vi "WIMDA data insert.vi"(8 "error in (no error)":errorcluster, 11 "WIMDA-data":T1) -> (0 "error out":errorcluster)   [LabVIEW 2016, in "AIRMAR WeatherCaster.lvlib"]
uses:
  AIRMAR WeatherCaster.lvlib
  NMEA_WIMDA-data.ctl
  <vilib>/addons/database/Auxilliary.llb/DB Tools Column Info.ctl
  <vilib>/addons/database/Auxilliary.llb/DB Tools DataTypes.ctl
  <vilib>/addons/database/NI_Database_API.lvlib
  <vilib>/Utility/VariantDataType/VariantType.lvlib
panel:
  in  "data in":T2
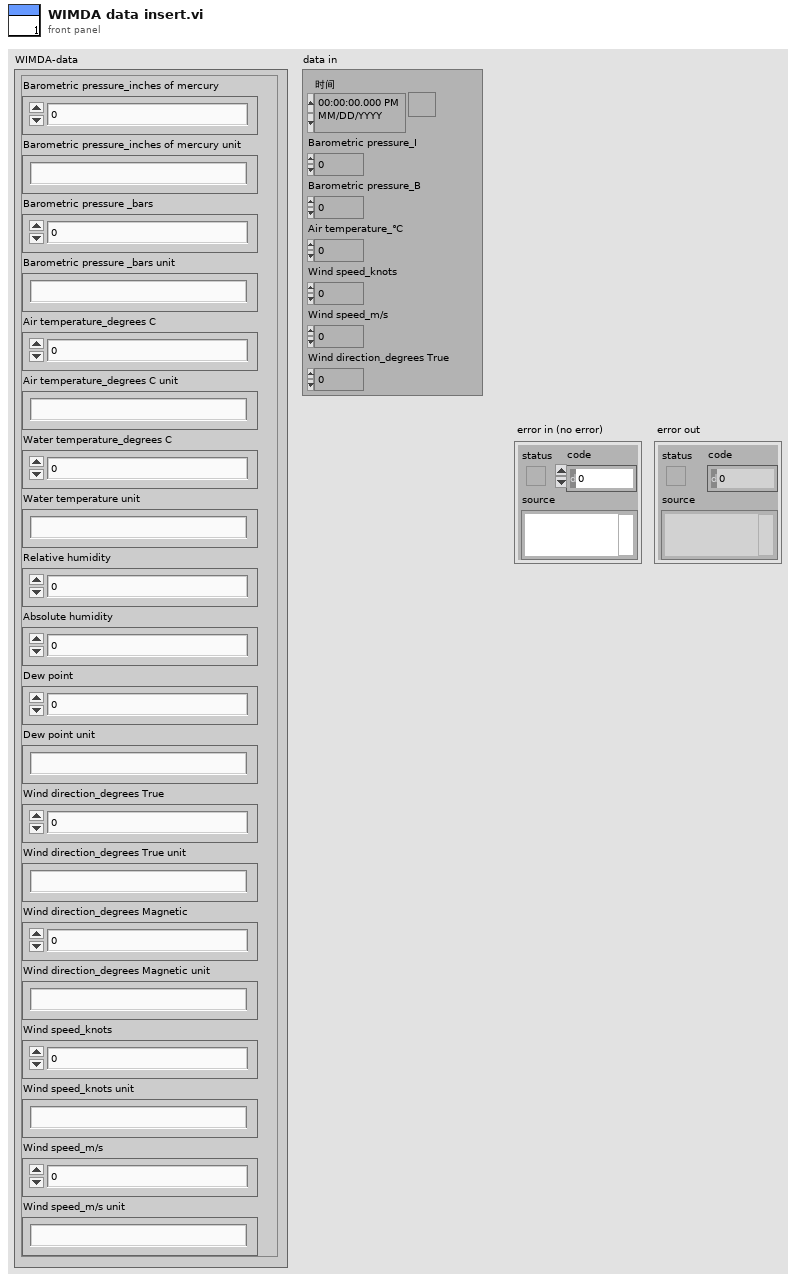
[diagram p1: front panel]
types:
  T1 = typedef "AIRMAR WeatherCaster.lvlib/NMEA_WIMDA-data.ctl" = cluster{"Barometric pressure_inches of mercury":dbl, "Barometric pressure_inches of mercury unit":string, "Barometric pressure _bars":dbl, "Barometric pressure _bars unit":string, "Air temperature_degrees C":dbl, "Air temperature_degrees C unit":string, "Water temperature_degrees C":dbl, "Water temperature unit":string, "Relative humidity":dbl, "Absolute humidity":dbl, "Dew point":dbl, "Dew point unit":string, "Wind direction_degrees True":dbl, "Wind direction_degrees True unit":string, "Wind direction_degrees Magnetic":dbl, "Wind direction_degrees Magnetic unit":string, "Wind speed_knots":dbl, "Wind speed_knots unit":string, "Wind speed_m/s":dbl, "Wind speed_m/s unit":string}
  T2 = cluster{"时间":timestamp, "Barometric pressure_I":dbl, "Barometric pressure_B":dbl, "Air temperature_℃":dbl, "Wind speed_knots":dbl, "Wind speed_m/s":dbl, "Wind direction_degrees True":dbl}
  T3 = typedef "NI_Database_API.lvlib/DB Tools Column Info.ctl" = cluster{"column name":string, "data type":T4, "size":i32, "allow null?":bool}
  T4 = typedef "NI_Database_API.lvlib/DB Tools DataTypes.ctl" = enum16{"String", "Long (I32)", "Single (SGL)", "Double (DBL)", "Date/Time", "Binary"}
  T5 = typedef "VariantType.lvlib/Type.ctl" = enum8{"Invalid Type", "Void", "I8", "I16", "I32", "I64", "U8", "U16", "U32", "U64", "Single Float", "Double Float", "Extended Float", "Single Complex", "Double Complex", "Extended Complex", "Enum U8", "Enum U16", "Enum U32", "Enum U64", "Single Float With Unit", "Double Float With Unit", "Extended Float With Unit", "Single Complex with Unit", "Double Complex with Unit", "Extended Complex with Unit", "Boolean", "String", "Path", "Picture", "Tag", "Array", "Cluster", "Variant", "LV Variant", "Waveform", "Timestamp", "Digital Waveform", "Digital Data", "ExpressData", "Refnum", "External Data", "VI", "Poly VI", "LabVIEW Class Instance", "Fixed Point"}
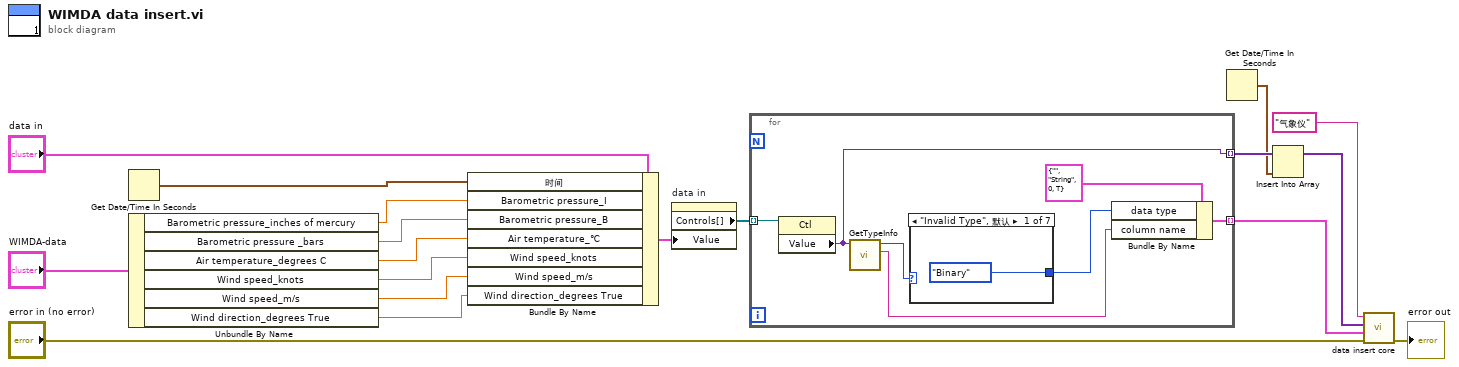
[diagram p0: block diagram]
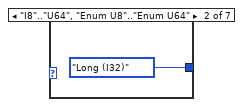
[diagram p2: hidden frame]
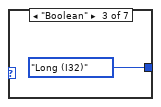
[diagram p3: hidden frame]
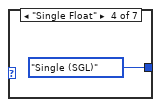
[diagram p4: hidden frame]
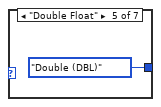
[diagram p5: hidden frame]
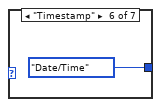
[diagram p6: hidden frame]
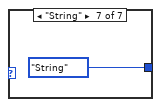
[diagram p7: hidden frame]
diagram:
  n1 = Get Date/Time In Seconds() -> (seconds since 1Jan1904=w8:timestamp)
  n2 = Unbundle By Name("WIMDA-data") -> ("Barometric pressure_inches of mercury"=w7:dbl, "Barometric pressure _bars"=w6:dbl, "Air temperature_degrees C"=w5:dbl, "Wind speed_knots"=w4:dbl, "Wind speed_m/s"=w3:dbl, "Wind direction_degrees True"=w2:dbl)
  n3 = Bundle By Name(cluster="data in", "时间"=w8, "Barometric pressure_I"=w7, "Barometric pressure_B"=w6, "Air temperature_℃"=w5, "Wind speed_knots"=w4, "Wind speed_m/s"=w3, "Wind direction_degrees True"=w2) -> (w1:T2)
  n4 = property on="data in" class="Clust (严格)"("Value"=w1) -> ("Controls[]"=w18:refnum<vi>[])  [unwired: 2 in, 2 out]
  n5 = for {
    tunnel: w18 -> [w25] mode=indexing
    tunnel: [w19] -> w17 mode=indexing
    tunnel: [w20] -> w12 mode=indexing
    n6 = property class="Ctl"(reference=w25) -> ("Value"=w19:variant)  [unwired: 1 in, 2 out]
    n7 = call <vilib>:"GetTypeInfo.vi"("Variant"=w19) -> ("Name"=w23:string, "Type Enum"=w22:T5)  [unwired: 6 in, 3 out]
    n8 = case shown="\"Invalid Type\", 默认" w22 {
      tunnel: [DB_Tools_DataTypes."Binary" ("data type") DB_Tools_DataTypes."Long (I32)" ("data type") DB_Tools_DataTypes."Long (I32)" ("data type") DB_Tools_DataTypes."Single (SGL)" ("data type") DB_Tools_DataTypes."Double (DBL)" ("data type") DB_Tools_DataTypes."Date/Time" ("data type") DB_Tools_DataTypes."String" ("data type")] -> w21
      frame "Invalid Type", Default {
      }
      frame "I8".."U64", "Enum U8".."Enum U64" {
      }
      frame "Boolean" {
      }
      frame "Single Float" {
      }
      frame "Double Float" {
      }
      frame "Timestamp" {
      }
      frame "String" {
      }
    }
    n9 = Bundle By Name(cluster=T3 {"column name"="", "data type"=enum."String", "size"=0, "allow null?"=TRUE} ("column information"), "data type"=w21, "column name"=w23) -> (w20:T3)
  }
  n10 = Get Date/Time In Seconds() -> (seconds since 1Jan1904=w16:timestamp)
  n11 = Insert Into Array(array=w17, new element=w16) -> (w15:variant[])  [unwired: 1 in]
  n12 = call "data insert core.vi"("error in (no error)"="error in (no error)", "column information"=w12, "data"=w15, "table"="气象仪") -> ("error out"=→"error out":errorcluster)  [unwired: 7 in]
